vi "CreateRootCore.vi"(9 "InnerLayers":T1[](array[typedef]), 10 "Alias":string, 11 "Root":refnum<class "Actor.lvclass">) -> ()   [LabVIEW 2020, in "jettl.lvlib"]
uses:
  jettl.lvlib
  Msg/Msg.lvclass
  Base/Actor/Actor.lvclass
  C:/Users/nathan.davis/Desktop/personal/jettl-harness/repos/jettl/src/jettl/jettl/Base/Actor/Actor.lvclass
  C:/Users/nathan.davis/Desktop/personal/jettl-harness/repos/jettl/src/jettl/jettl/Actor/Actor.lvclass
  Actor/Actor.lvclass
  Lifecycle.ctl
  Msg.ctl
  MsgSet.ctl
  Unified.ctl
  PostSetup.ctl
  SpawnComponent.vi
  Base/Base.lvlib
  PreSetup.ctl
  Origin.ctl
  Metadata.ctl
  ActorMap.ctl
  Metadata/Metadata.lvclass
panel:
  in  "MsgDVR":refnum<data-value>
  in  "Actor in 2":refnum<class "Actor.lvclass">
  in  "Actors 2":refnum<class "Actor.lvclass">[](array[class])
  out "Actor out 2":refnum<class "Actor.lvclass">
  out "Actor out":refnum<class "Actor.lvclass">
  in  "Actor in":refnum<class "Actor.lvclass">
  in  "Actors":refnum<class "Actor.lvclass">[](array[class])
  in  "ActorAlias":string
  in  "Error in 2":errorcluster
  out "Error out 2":errorcluster
  in  "Teller 2":T2 {"AbsoluteTime" format="%<%x %.3X>T"}
  out "ConcreteActor 4":refnum<class "Actor.lvclass">
  in  "ConcreteActor 3":refnum<class "Actor.lvclass">
  in  "Error in":errorcluster
  out "Error out":errorcluster
  in  "Error":errorcluster
  in  "Teller":T2 {"AbsoluteTime" format="%<%x %.3X>T"}
  in  "Actor 2":refnum<class "Actor.lvclass">
  out "ConcreteActor":refnum<class "Actor.lvclass">
  in  "ConcreteActor 2":refnum<class "Actor.lvclass">
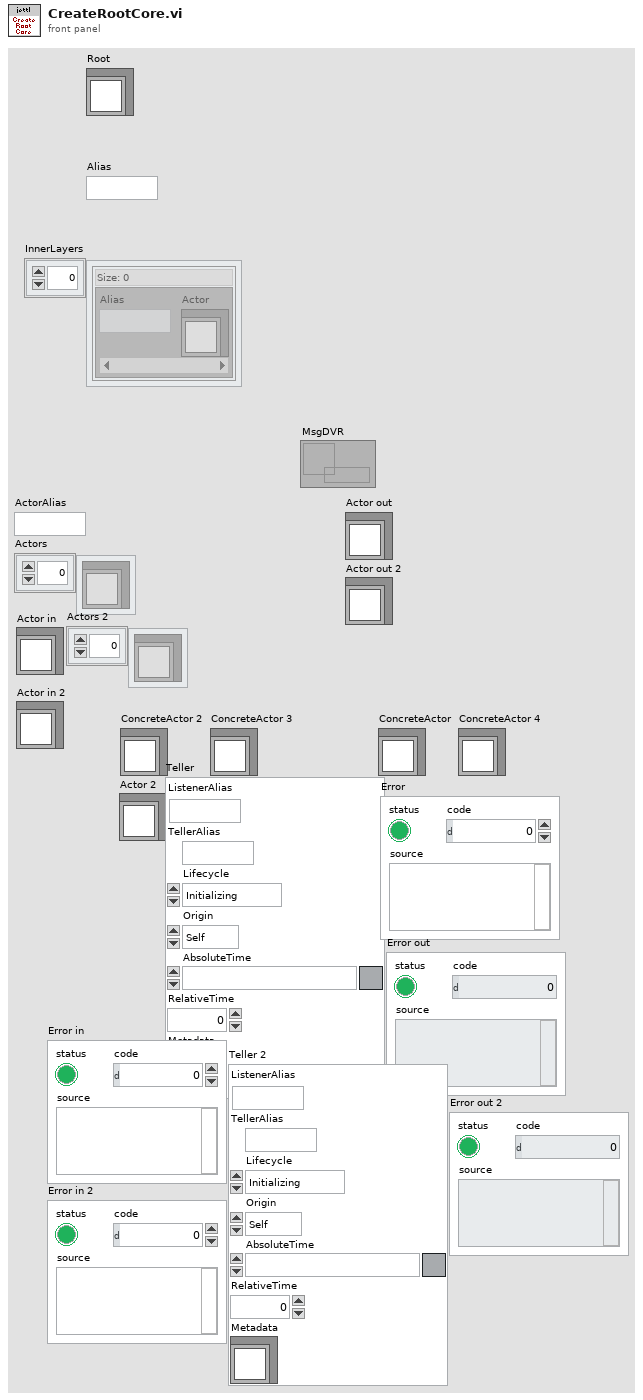
[diagram p1: front panel]
types:
  T1 = typedef "jettl.lvlib/ActorMap.ctl" = map{string, refnum<class "Actor.lvclass">}
  T2 = typedef "jettl.lvlib/Metadata.ctl" = cluster{"ListenerAlias":string, "TellerAlias":string, "Lifecycle":T3, "Origin":T4, "AbsoluteTime":timestamp, "RelativeTime":dbl, "Metadata":refnum<class "Metadata.lvclass">}
  T3 = typedef "jettl.lvlib/Lifecycle.ctl" = enum16{"Initializing", "SettingUp", "Starting", "Running", "Stopping", "TearingDown", "Terminated"}
  T4 = typedef "jettl.lvlib/Origin.ctl" = enum16{"Self", "Parent", "Child"}
  T5 = typedef "jettl.lvlib/PostSetup.ctl" = cluster{"Error":errorcluster}
  T6 = typedef "jettl.lvlib/Unified.ctl" = cluster{"Alias":string, "MsgSet":T7, "Root":bool, "Leaf":bool, "MsgDVREvent":refnum<user-event>, "EventRegRef":refnum<event-registration>, "PreSetupQueue":refnum<queue>, "BeginSetupQueue":refnum<queue>, "PostSetupQueue":refnum<queue>, "VIRef":refnum<vi>, "DestroyQueue":refnum<queue>}
  T7 = typedef "jettl.lvlib/MsgSet.ctl" = set{refnum<class "Msg.lvclass">}
  T8 = typedef "jettl.lvlib/Base.ctl" = cluster{"State":T9, "SelfUnified":T6, "ParentUnified":T6, "ChildUnifiedMap":T10}
  T9 = typedef "jettl.lvlib/State.ctl" = cluster{"Lifecycle":T3}
  T10 = typedef "jettl.lvlib/ChildUnifiedMap.ctl" = map{string, T6}
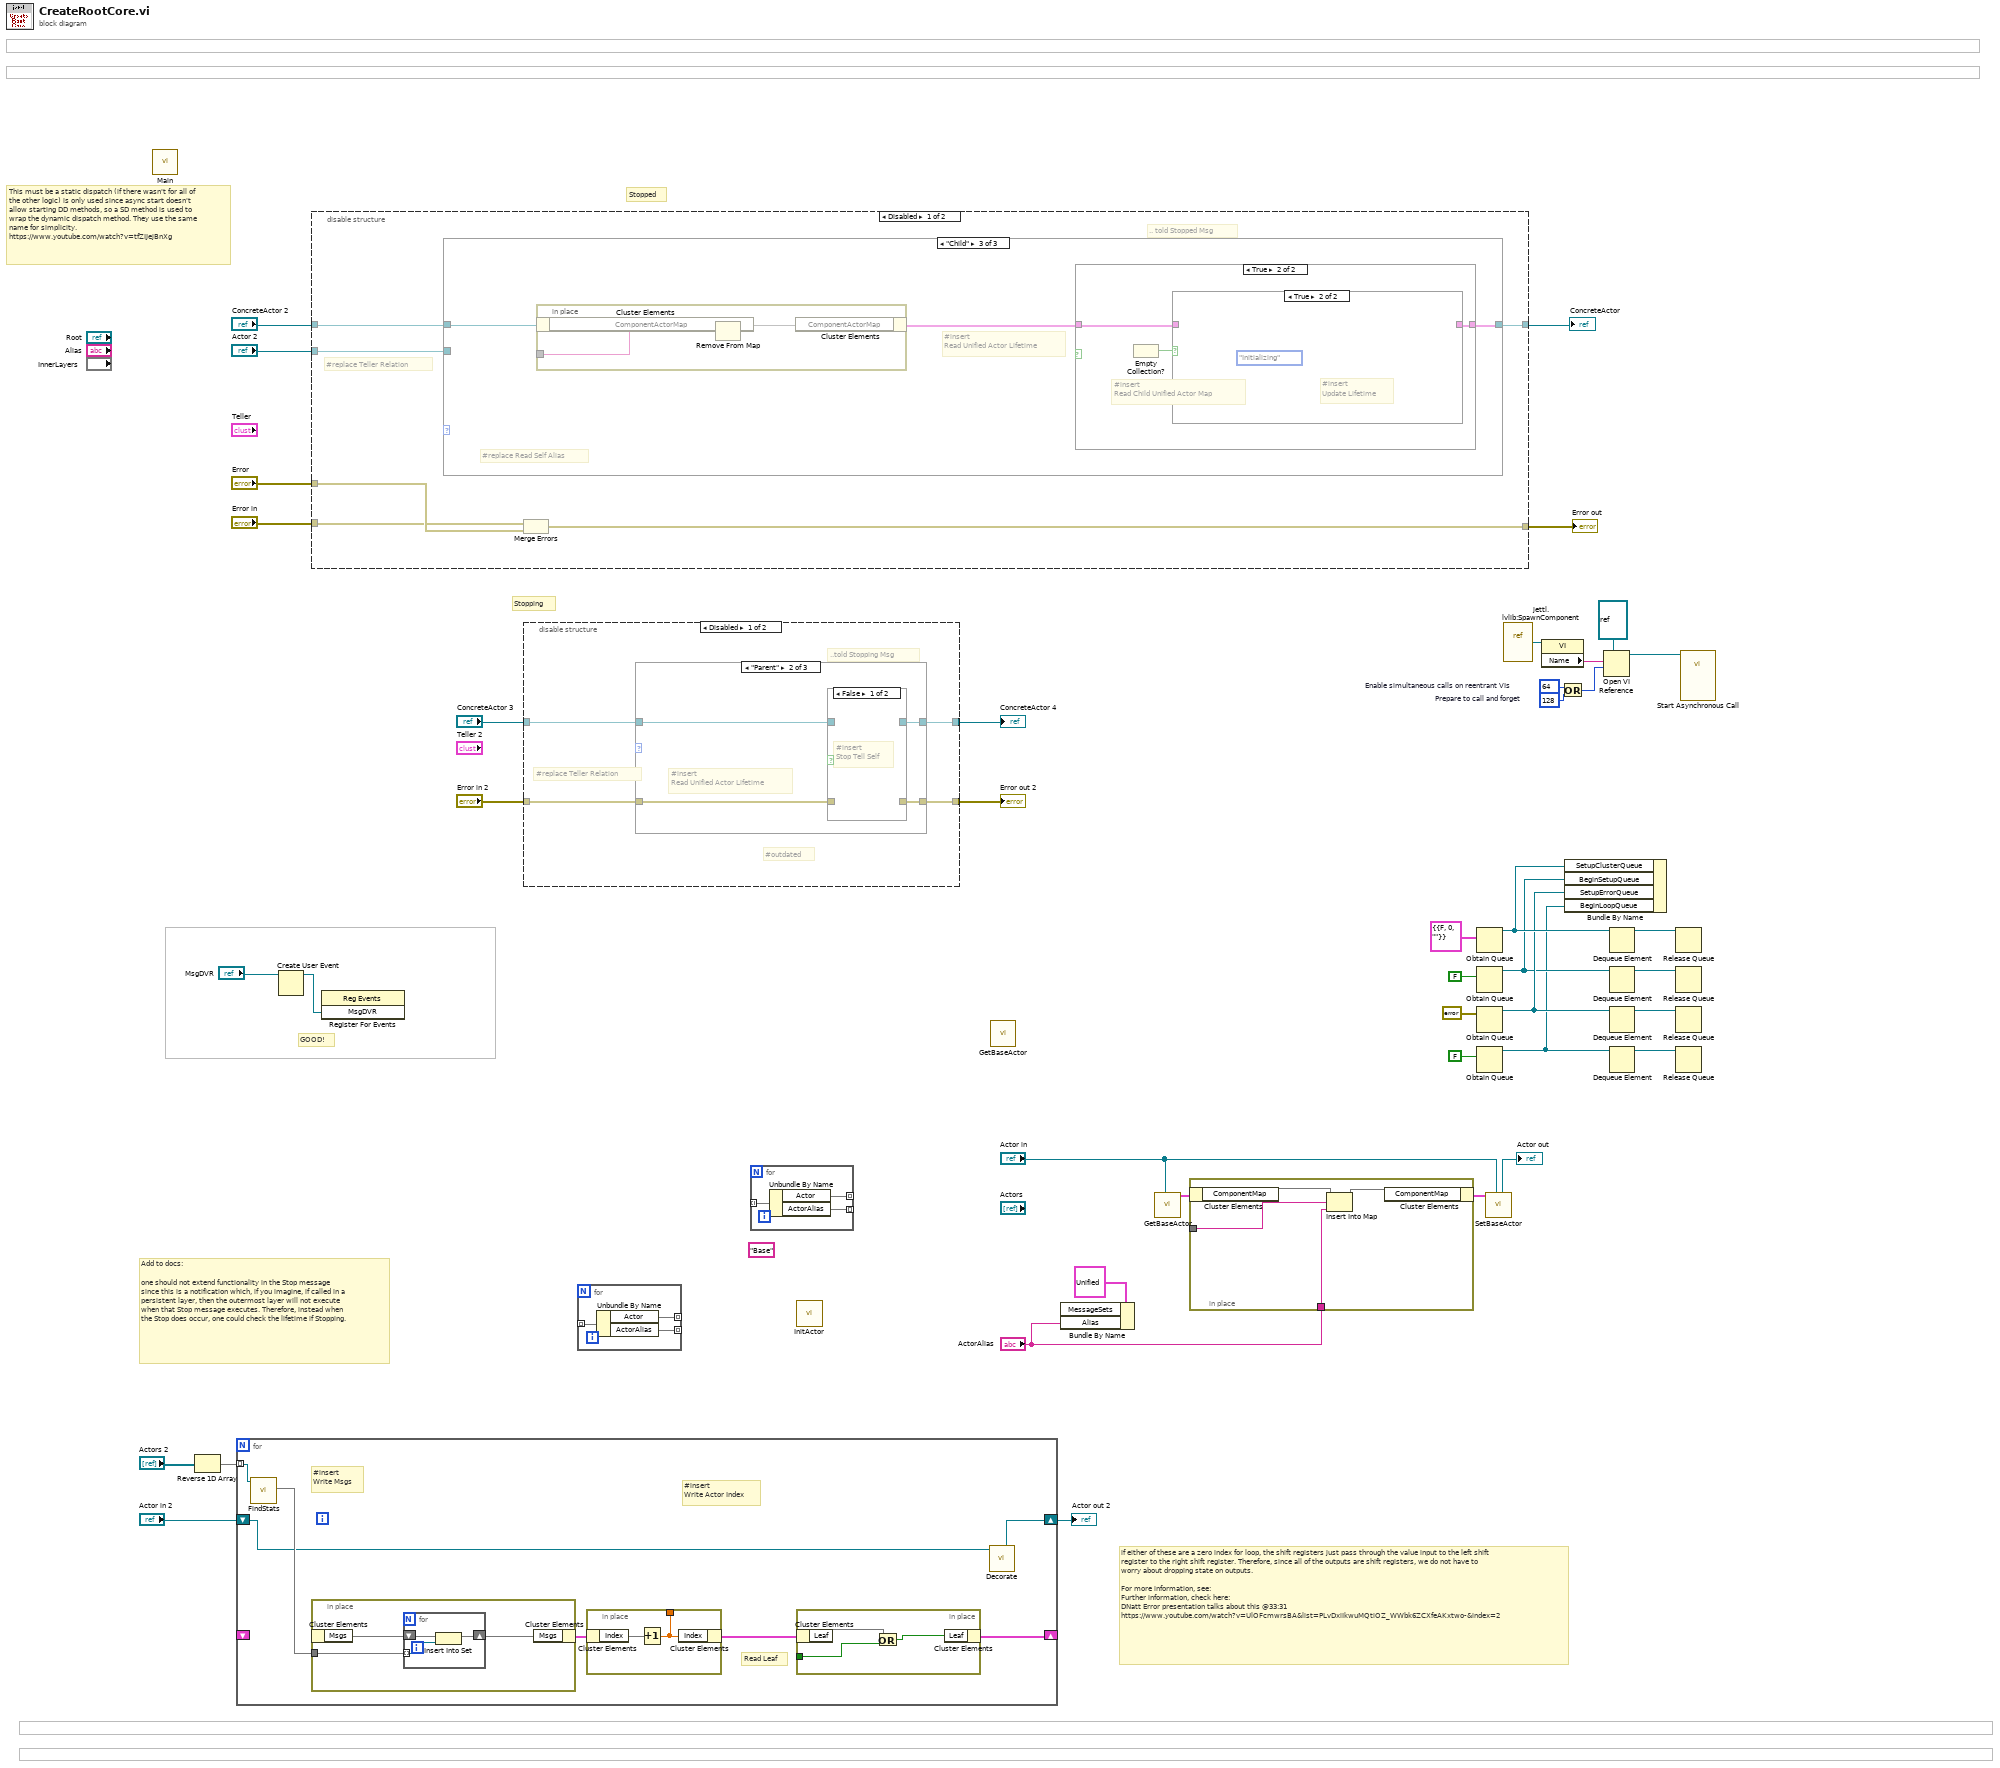
[diagram p0: block diagram]
diagram:
  w6 = 64  # Enable simultaneous calls on reentrant VIs
  w7 = 128  # Prepare to call and forget
  (unwired) "Base"
  # "GOOD!"
  # "if either of these are a zero index for loop, the shift registers just pass through the value input to the left shift register to the right shift register. Therefore, since all of the outputs are shift registers, we do not have to worry about dropping state on outputs.\n\nFor more information, see:\nFurther information, check here:\nDNatt Error presentation talks about this @33:31\nhttps://www.youtube.com/watch?v=UlOFcmwrsBA&list=PLvDxiIkwuMQtiOZ_WWbk6ZCXfeAKxtwo-&index=2"
  # "Add to docs:\n\none should not extend functionality in the Stop message since this is a notification which, if you imagine, if called in a persistent layer, then the outermost layer will not execute when that Stop message executes. Therefore, instead when the Stop does occur, one could check the lifetime if Stopping."
  # "Stopped"
  # "Stopping"
  # "This must be a static dispatch (if there wasn't for all of the other logic) is only used since async start doesn't allow starting DD methods, so a SD method is used to wrap the dynamic dispatch method. They use the same name for simplicity.\nhttps://www.youtube.com/watch?v=tfZIJejBnXg"
  n1 = call-dynamic "Main.vi"() -> ()  [unwired: 12 in]
  n2 = Reverse 1D Array(array="Actors 2") -> (reversed array=w29:refnum<class "Actor.lvclass">[])
  n3 = for {
    tunnel: w29 -> [w52] mode=indexing
    shift-right: [w47] -> w28
    shift-left: "Actor in 2" -> [w45]
    shift-right: [w53] -> w25
    shift-left: _ -> [_]
    # "#insert\nWrite Actor Index"
    # "#insert\nWrite Msgs"
    # "Read Leaf"
    n4 = call-dynamic "FindStats.vi"(11:w52) -> (2:w54)  [unwired: 9 in, 1 out]
    n5 = in-place {
      in-place-border: w54 -> [w62]
      n6 = in-place-cluster #1() -> ("Msgs"=w61)  [unwired: 1 in]
      n7 = for {
        shift-right: [w64] -> w60
        shift-left: w61 -> [w65]
        tunnel: w62 -> [w63] mode=indexing
        n8 = Insert Into Set(10:w63, 11:w65) -> (3:w64:set{refnum<class "Message.lvclass">})  [unwired: 1 out]
      }
      n9 = in-place-cluster #1("Msgs"=w60) -> (w50:cluster{})
    }
    n10 = in-place {
      in-place-border: [w58] -> w48
      n11 = in-place-cluster #2(w50) -> ("Index"=w59)
      n12 = Increment(x=w59) -> (x+1=w58:dbl)
      n13 = in-place-cluster #2("Index"=w58) -> (w49:cluster{})
    }
    n14 = in-place {
      in-place-border: [w55] -> w51
      n15 = in-place-cluster #3(w49) -> ("Leaf"=w57)
      n16 = Or(x=w57, y=w55) -> (x .or. y?=w56:bool)
      n17 = in-place-cluster #3("Leaf"=w56) -> (w53:cluster{})
    }
    n18 = call-dynamic "Decorate.vi"("Actor"=w45) -> (5:"Actor"=w47:refnum<class "Actor.lvclass">, 7:"Actor"=w46:refnum<class "Actor.lvclass">)  [unwired: 9 in]
  }
  "Actor out 2" <- w28
  n19 = Create User Event(user event datatype="MsgDVR") -> (user event=w1:refnum<user-event>)  [unwired: 1 in, 1 out]
  n20 = disable-structure shown="Disabled" {
    disable-tunnel: [w71 w89] -> w44
    disable-tunnel: "ConcreteActor 2" -> [w70 w89]
    disable-tunnel: "Actor 2" -> [w69 _]
    disable-tunnel: "Error" -> [w68 _]
    disable-tunnel: "Error in" -> [w67 w90]
    disable-tunnel: [w66 w90] -> w39
    frame Disabled {
      # "#replace Teller Relation"
      # ".. told Stopped Msg"
      n21 = case shown="\"Child\"" {
        selector: _ -> [_ _ _]
        tunnel: w70 -> [w72 w73 w75]
        tunnel: [w72 w73 w77] -> w71
        tunnel: w69 -> [_ _ w76]
        frame "Self" {
          # "Case will not fundamentally execute"
        }
        frame "Parent" {
          # "Case will not fundamentally execute"
        }
        frame "Child" {
          # "#insert\nRead Unified Actor Lifetime"
          # "#replace Read Self Alias"
          n22 = in-place {
            in-place-border: [w80] -> _
            n23 = in-place-cluster #4(w75) -> ("ComponentActorMap"=w79)
            n24 = Remove From Map(11:w79) -> (3:w78:map{string, i32}, 10:w80:string)  [unwired: 2 out]
            n25 = in-place-cluster #4("ComponentActorMap"=w78) -> (w74:cluster{})
          }
          n26 = case shown="True" {
            selector: _ -> [_ _]
            tunnel: w74 -> [w81 w82]
            tunnel: [w81 w84] -> w77
            frame False {
            }
            frame True {
              # "#insert\nRead Child Unified Actor Map"
              n27 = Empty Collection?() -> (0:w83:bool)  [unwired: 1 in]
              n28 = case shown="True" w83 {
                tunnel: [w85 w86] -> w84
                tunnel: w82 -> [w85 w87]
                frame False {
                }
                frame True {
                  w88 = Lifecycle."Initializing" ("Lifetime")
                  # "#insert\nUpdate Lifetime"
                }
              }
            }
          }
        }
      }
      n29 = Merge Errors(w67, w68) -> (w66:errorcluster)
    }
    frame Enabled {
    }
  }
  "ConcreteActor" <- w44
  "Error out" <- w39
  n30 = register-events(w1) -> ()  [unwired: 2 in, 2 out]
  n31 = disable-structure shown="Disabled" {
    disable-tunnel: "ConcreteActor 3" -> [w94 w109]
    disable-tunnel: [w93 w109] -> w37
    disable-tunnel: "Error in 2" -> [w92 w108]
    disable-tunnel: [w91 w108] -> w35
    frame Disabled {
      # "#outdated"
      # "#replace Teller Relation"
      # "..told Stopping Msg"
      n32 = case shown="\"Parent\"" {
        selector: _ -> [_ _ _]
        tunnel: w94 -> [w96 w97 w107]
        tunnel: [w96 w100 w107] -> w93
        tunnel: w92 -> [w95 w99 w106]
        tunnel: [w95 w98 w106] -> w91
        frame "Self" {
          # "Case will not fundamentally execute"
        }
        frame "Parent" {
          # "#insert\nRead Unified Actor Lifetime"
          n33 = case shown="False" {
            selector: _ -> [_ _]
            tunnel: [w103 w105] -> w100
            tunnel: w99 -> [w102 w104]
            tunnel: [_ w104] -> w98
            tunnel: w97 -> [w101 w105]
            frame False {
              # "#insert\nStop Tell Self"
            }
            frame True {
            }
          }
        }
        frame "Child" {
          # "Case will not fundamentally execute"
        }
      }
    }
    frame Enabled {
    }
  }
  "ConcreteActor 4" <- w37
  "Error out 2" <- w35
  n34 = for {
    tunnel: [w112] -> _ mode=indexing
    tunnel: [w111] -> _ mode=indexing
    tunnel: _ -> [w110] mode=indexing
    n35 = Unbundle By Name(w110) -> ("Actor"=w112, "ActorAlias"=w111)
  }
  n36 = for {
    tunnel: [w115] -> _ mode=indexing
    tunnel: [w114] -> _ mode=indexing
    tunnel: _ -> [w113] mode=indexing
    n37 = Unbundle By Name(w113) -> ("Actor"=w115, "ActorAlias"=w114)
  }
  n38 = call "InitActor.vi"() -> ()  [unwired: 11 in, 1 out]
  n39 = call-dynamic "GetBaseActor.vi"() -> ()  [unwired: 11 in, 1 out]
  n40 = Bundle By Name(cluster=T6 {"Alias"="", "MsgSet"={}, "Root"=FALSE, "Leaf"=FALSE, "MsgDVREvent"=refnum, "EventRegRef"=refnum, "PreSetupQueue"=refnum, "BeginSetupQueue"=refnum, "PostSetupQueue"=refnum, "VIRef"=refnum, "DestroyQueue"=refnum} ("Attributes"), "Alias"="ActorAlias") -> (w30:T6)  [unwired: 1 in]
  n41 = call-dynamic "GetBaseActor.vi"("Actor"="Actor in") -> ("BaseActor"=w13:T8)  [unwired: 10 in]
  n42 = in-place {
    in-place-border: "ActorAlias" -> [w119]
    in-place-border: [w118] -> w11
    n43 = in-place-cluster #5(w13) -> ("ComponentMap"=w117)
    n44 = Insert Into Map(map in=w117, value=w119) -> (key=w118:string, map out=w116:map{string, string})  [unwired: 2 out]
    n45 = in-place-cluster #5("ComponentMap"=w116) -> (w12:T8)
  }
  n46 = Obtain Queue(element data type=T5 {"Error"={"status"=FALSE, "code"=0, "source"=""}} ("PreSetup")) -> (queue out=w21:refnum<queue>)  [unwired: 4 in, 2 out]
  n47 = Obtain Queue(element data type=FALSE) -> (queue out=w16:refnum<queue>)  [unwired: 4 in, 2 out]
  n48 = Obtain Queue(element data type=errorcluster {"status"=FALSE, "code"=0, "source"=""} ("Error")) -> (queue out=w17:refnum<queue>)  [unwired: 4 in, 2 out]
  n49 = Obtain Queue(element data type=FALSE) -> (queue out=w15:refnum<queue>)  [unwired: 4 in, 2 out]
  n50 = call-dynamic "SetBaseActor.vi"("Actor"="Actor in", "BaseActor"=w12) -> ("Actor"=→"Actor out":refnum<class "Actor.lvclass">)  [unwired: 9 in]
  n51 = vi-ref "jettl.lvlib:SpawnComponent.vi"() -> (w9:refnum<vi>)
  n52 = property class="VI"(reference=w9) -> ("Name"=w10:string)  [unwired: 1 in, 2 out]
  n53 = Or(x=w6, y=w7) -> (x .or. y?=w5:i32)
  n54 = Bundle By Name("SetupClusterQueue"=w21, "BeginSetupQueue"=w16, "SetupErrorQueue"=w17, "BeginLoopQueue"=w15) -> ()  [unwired: 1 in, 1 out]
  n55 = Open VI Reference(type specifier VI Refnum (for type only)=refnum<vi> refnum, vi path=w10, options=w5) -> (vi reference=w4:refnum<vi>)  [unwired: 3 in, 1 out]
  n56 = Dequeue Element(queue=w21) -> (queue out=w22:refnum<queue>)  [unwired: 2 in, 3 out]
  n57 = Dequeue Element(queue=w16) -> (queue out=w24:refnum<queue>)  [unwired: 2 in, 3 out]
  n58 = Dequeue Element(queue=w17) -> (queue out=w20:refnum<queue>)  [unwired: 2 in, 3 out]
  n59 = Dequeue Element(queue=w15) -> (queue out=w3:refnum<queue>)  [unwired: 2 in, 3 out]
  n60 = Release Queue(queue=w22) -> ()  [unwired: 2 in, 3 out]
  n61 = Release Queue(queue=w24) -> ()  [unwired: 2 in, 3 out]
  n62 = Release Queue(queue=w20) -> ()  [unwired: 2 in, 3 out]
  n63 = Release Queue(queue=w3) -> ()  [unwired: 2 in, 3 out]
  n64 = call-by-ref "Start Asynchronous Call"(reference=w4) -> ()  [unwired: 13 in, 2 out]
